vi "Main.vi"(8 "error in":errorcluster, 11 "Analog Signal in":refnum<class "Analog Signal.lvclass">) -> (0 "error out":errorcluster, 3 "Analog Signal out":refnum<class "Analog Signal.lvclass">)   [LabVIEW 2023, in "Analog Signal.lvclass"]
doc: "The <b>Queued Message Handler</b> of the Worker that owns this VI."
uses:
  Analog Signal.lvclass
  C:/Program Files (x86)/National Instruments/LabVIEW 2023/vi.lib/addons/_Workers/Library/Classes/Worker/Worker.lvclass
  Support/Signal Type.ctl
  Support/Signal Config.ctl
  Support/Sampling Config.ctl
  Initialization Data.ctl
  Response Cases.ctl
  <vilib>/addons/_Workers/Library/Case Label.ctl
  Analog Signal.lvclass/Analog Signal.ctl
  rql_Set Sampling Config.ctl
  rqp_Set Signal Config.ctl
  rqp_Set Sampling.ctl
  rqp_Insert to Subpanel.ctl
  rsp_Acquisition.ctl
  <vilib>/Utility/error.llb/Error Cluster From Error Code.vi
  <vilib>/ErrorRing/Error Ring.xnode
  Message Pump/Message Pump.lvclass
  <vilib>/addons/_Workers/Library/Workers.lvlib
panel:
  out "Response Cases.Sampling_Config":T1={"Fs"=1000.0, "#s"=1000.0} {"Fs" format="%.2p"}
  out "Response Cases.Signal_Config":T2={"offset"=0.0, "frequency"=10.0, "amplitude"=1.0} {"amplitude" format="%#_13g"; "frequency" format="%#_13g"; "offset" format="%0.2p"}
  out "Response Cases.Signal Type":T3
  out "Waveform Chart":waveform(dbl)(graph)
  # "Analog Signal"
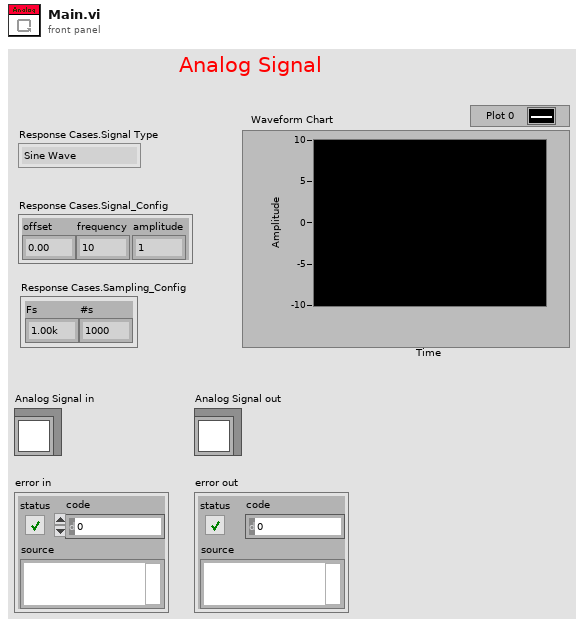
[diagram p1: front panel]
types:
  T1 = typedef "Analog Signal.lvclass/Sampling Config.ctl" = cluster{"Fs":dbl, "#s":dbl}
  T2 = typedef "Analog Signal.lvclass/Signal Config.ctl" = cluster{"offset":dbl, "frequency":dbl, "amplitude":dbl}
  T3 = typedef "Analog Signal.lvclass/Signal Type.ctl" = enum16{"Sine Wave", "Square Wave"}
  T4 = enum32{"Invalid", "Standard", "Closed", "Hidden", "Minimized", "Maximized"}
  T5 = typedef "Analog Signal.lvclass/Initialization Data.ctl" = cluster{"Response Cases":T6}
  T6 = typedef "Analog Signal.lvclass/Response Cases.ctl" = cluster{"Signal Type":T3, "Signal_Config":T2, "Sampling_Config":T1, "Acquisition":T7}
  T7 = typedef "Workers.lvlib/Case Label.ctl" = string
  T8 = typedef "Analog Signal.lvclass/rql_Set Sampling Config.ctl" = cluster{"Sampling_Config":T1}
  T9 = typedef "Analog Signal.lvclass/rqp_Set Signal Config.ctl" = cluster{"Signal_Config":T2, "Signal Type":T3}
  T10 = typedef "Analog Signal.lvclass/rqp_Set Sampling.ctl" = cluster{"Sampling_Config":T1}
  T11 = typedef "Analog Signal.lvclass/rqp_Insert to Subpanel.ctl" = cluster{"Sub Panel Ref":refnum<vi>}
  T12 = typedef "Analog Signal.lvclass/rsp_Acquisition.ctl" = cluster{"Waveform":waveform(dbl)}
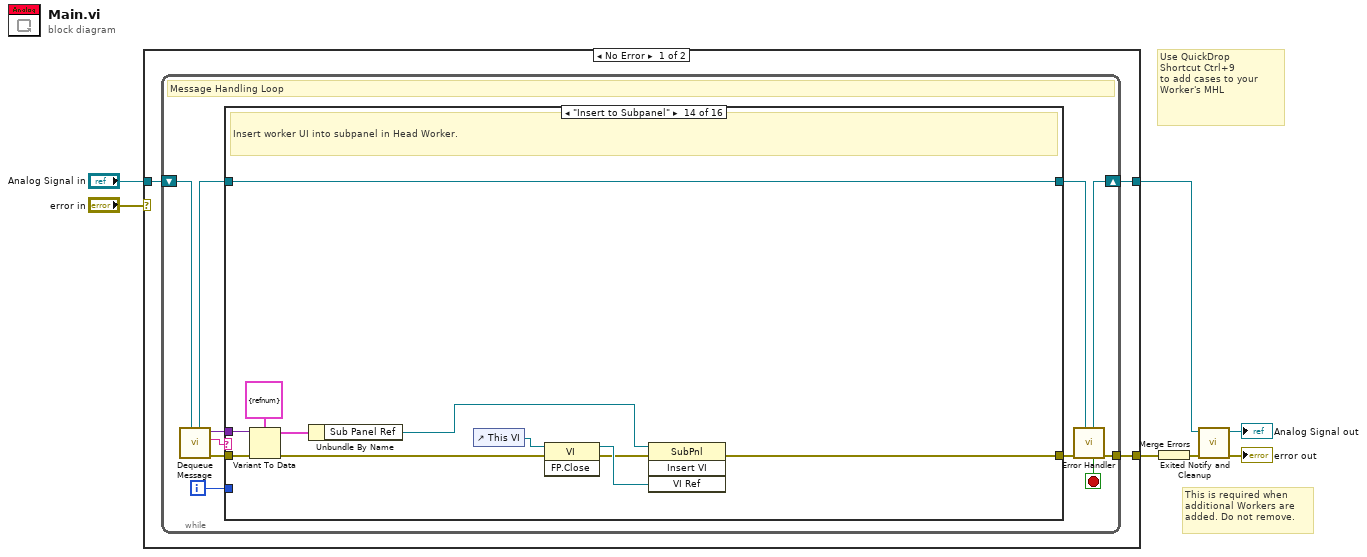
[diagram p0: block diagram]
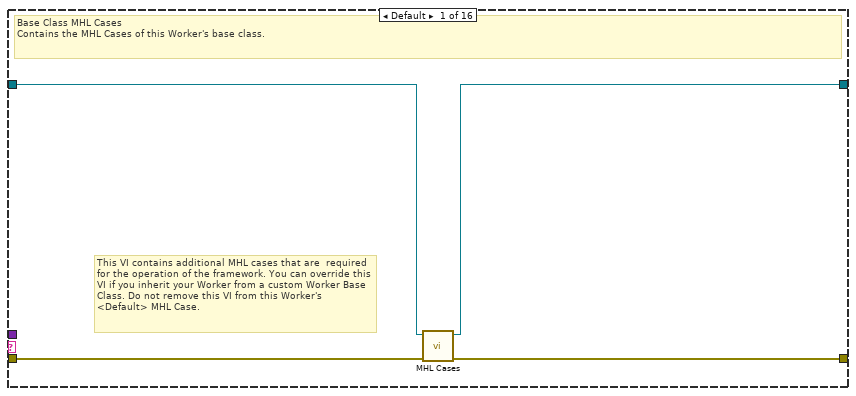
[diagram p2: hidden frame]
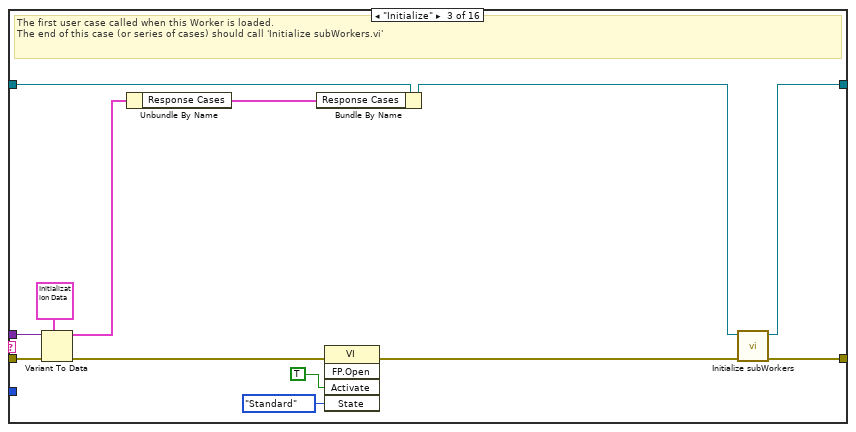
[diagram p4: hidden frame]
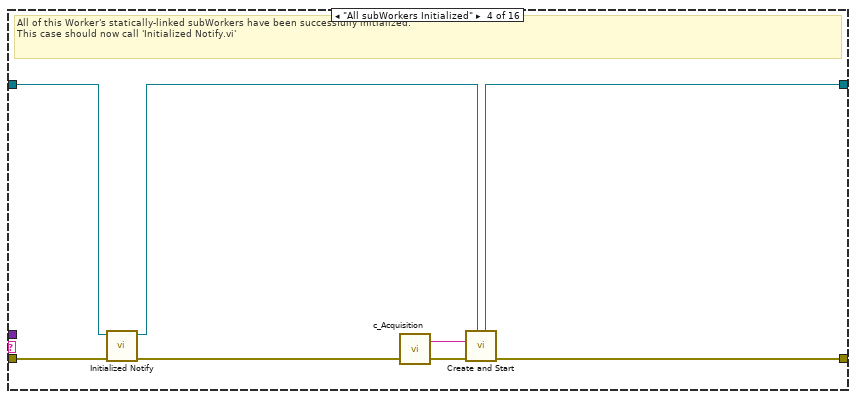
[diagram p5: hidden frame]
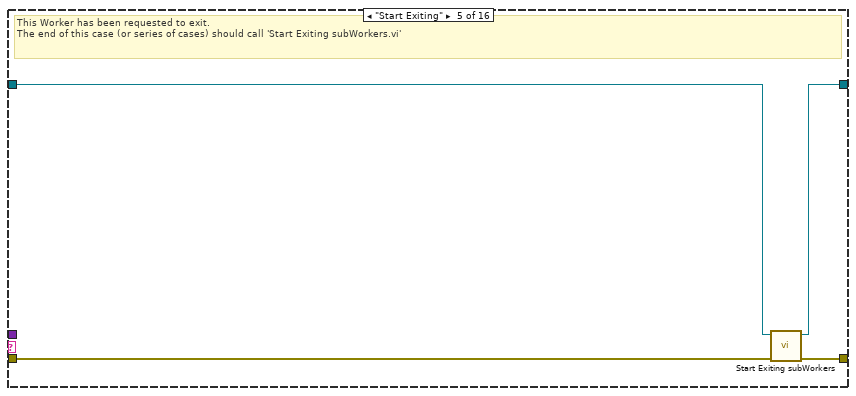
[diagram p6: hidden frame]
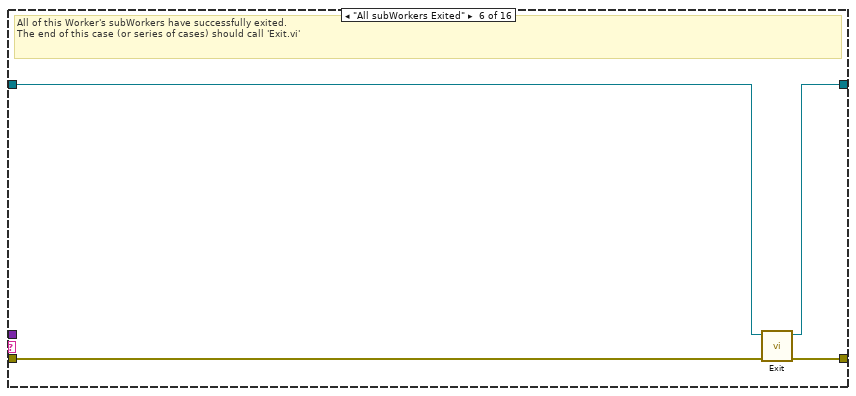
[diagram p7: hidden frame]
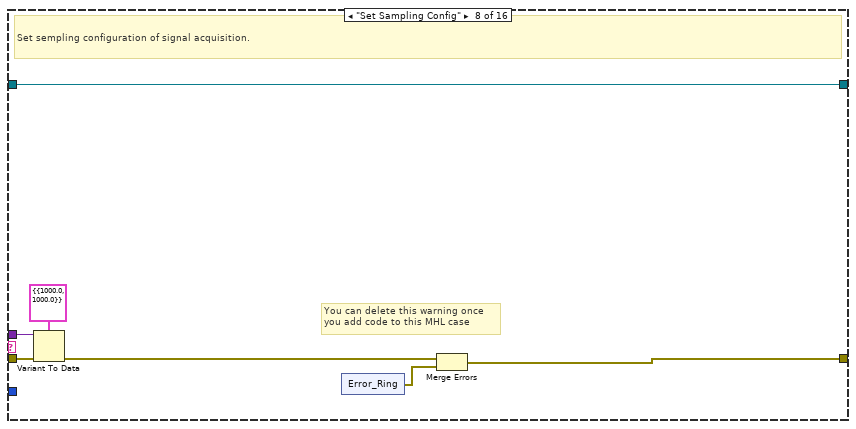
[diagram p9: hidden frame]
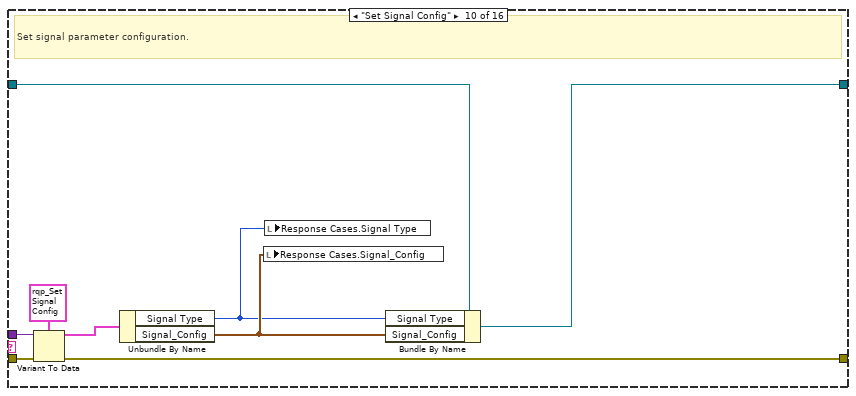
[diagram p11: hidden frame]
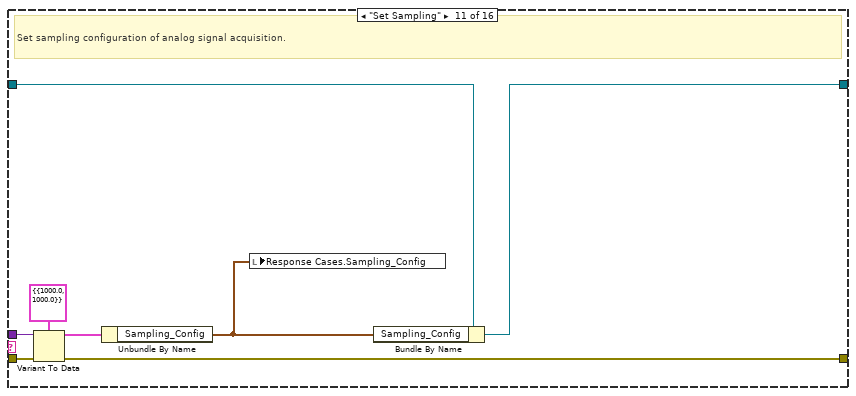
[diagram p12: hidden frame]
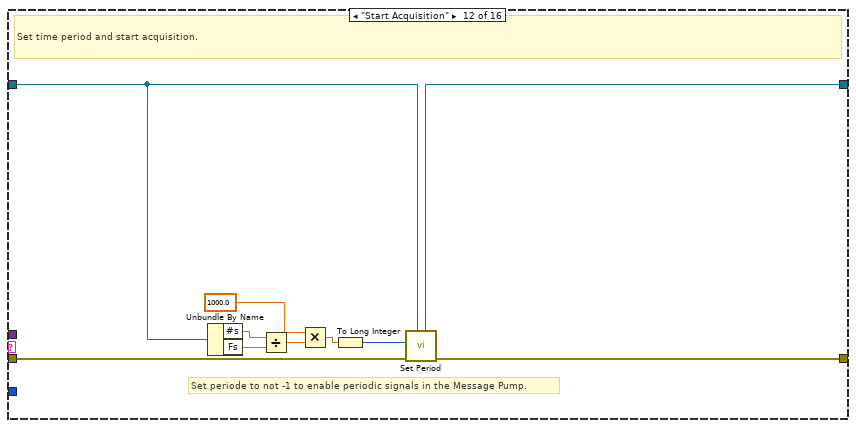
[diagram p13: hidden frame]
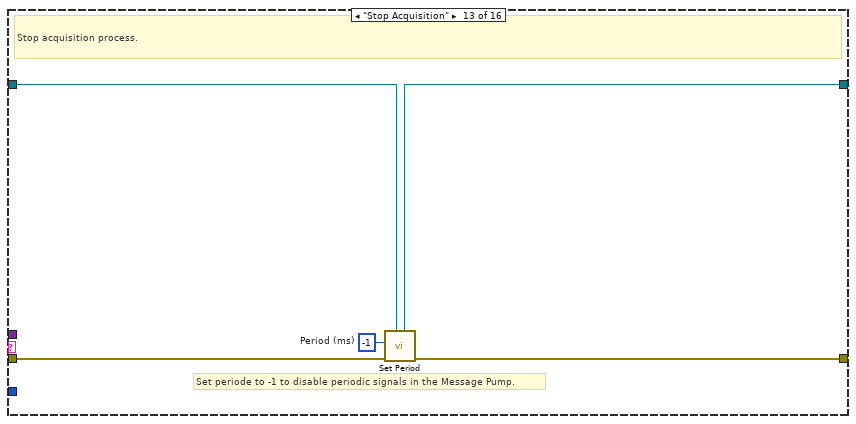
[diagram p14: hidden frame]
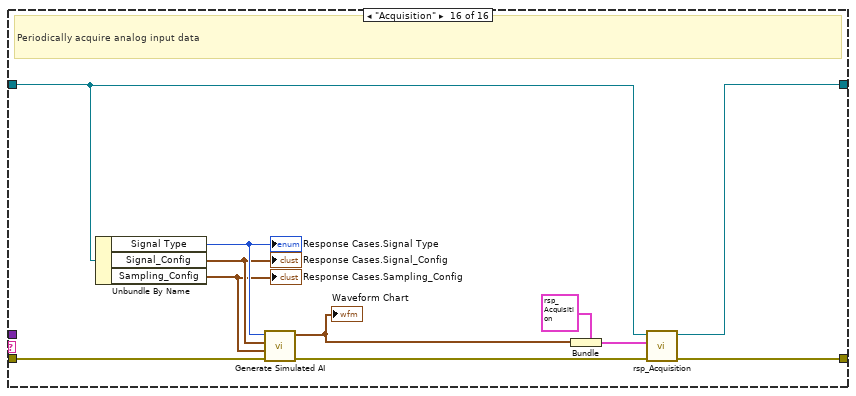
[diagram p16: hidden frame]
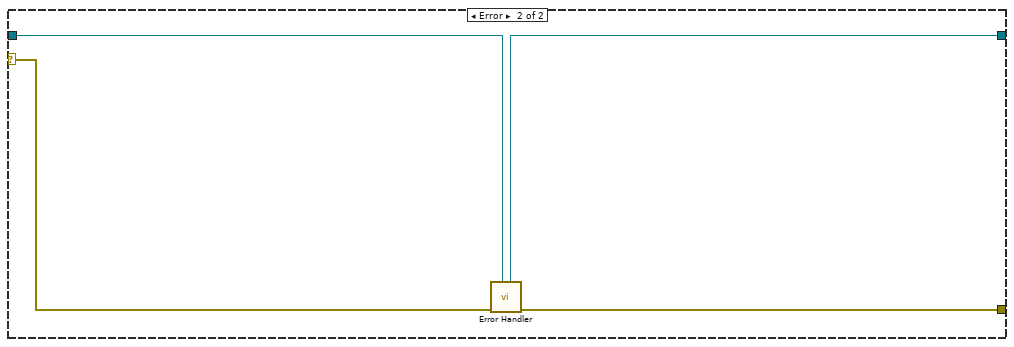
[diagram p17: hidden frame]
diagram:
  # "Use QuickDrop\nShortcut Ctrl+9\nto add cases to your\nWorker's MHL"
  # "This is required when additional Workers are added. Do not remove."
  n1 = case shown="No Error" "error in" {
    tunnel: "Analog Signal in" -> [w8 w129]
    tunnel: [w10 w130] -> w6
    tunnel: [w9 w128] -> w7
    selector: "error in" -> [_ w131]
    frame No Error {
      n2 = while {
        shift-right: [w19] -> w9
        shift-left: w8 -> [w21]
        tunnel: [w20] -> w10
        i -> [w12]
        stop <- w13 stop-if-true
        # "Message Handling Loop"
        n3 = call-dynamic "Dequeue Message.vi"("Worker"=w21) -> ("error out"=w18:errorcluster, "Case out"=w14:string, "Data out"=w11:variant, "Worker out"=w16:refnum<class "Analog Signal.lvclass">)  [unwired: 6 in, 1 out]
        n4 = case "Worker MHL Case Structure (DO NOT CHANGE LABEL NAME)" shown="\"Insert to Subpanel\"" w14 {
          tunnel: w18 -> [w25 w26 w38 w47 w48 w55 w57 w63 w71 w79 w88 w97 w100 w113 w116 w127]
          tunnel: [w24 w26 w40 w42 w51 w54 w57 w59 w71 w78 w87 w96 w99 w104 w116 w122] -> w17
          tunnel: w16 -> [w23 w27 w37 w46 w49 w53 w56 w64 w70 w80 w84 w95 w102 w114 w115 w121]
          tunnel: [w22 w27 w39 w44 w50 w52 w56 w64 w70 w75 w83 w98 w101 w114 w115 w120] -> w15
          tunnel: w12 -> [_ _ _ _ _ _ _ _ _ _ _ _ _ _ _ _]
          tunnel: w11 -> [_ _ w36 _ _ _ _ w60 _ w76 w85 _ _ w111 _ _]
          frame Default {
            # "This VI contains additional MHL cases that are  required for the operation of the framework. You can override this VI if you inherit your Worker from a custom Worker Base Class. Do not remove this VI from this Worker's <Default> MHL Case."
            # "Base Class MHL Cases\nContains the MHL Cases of this Worker's base class."
            n5 = call-dynamic "MHL Cases.vi"("error in"=w25, "Worker in"=w23) -> ("error out"=w24:errorcluster, "Worker out"=w22:refnum<class "Analog Signal.lvclass">)  [unwired: 8 in]
          }
          frame "------------ FRAMEWORK CASES -----------" {
            # "Start of Workers Framework Cases"
          }
          frame "Initialize" {
            # "The first user case called when this Worker is loaded.\nThe end of this case (or series of cases) should call 'Initialize subWorkers.vi'"
            n6 = Variant To Data(error in=w38, type=T5 {"Response Cases"={"Signal Type"=enum."Sine Wave", "Signal_Config"={"offset"=0.0, "frequency"=10.0, "amplitude"=1.0}, "Sampling_Config"={"Fs"=1000.0, "#s"=1000.0}, "Acquisition"=""}} ("Cluster"), Variant=w36) -> (data=w34:T5, error out=w29:errorcluster)
            n7 = Unbundle By Name(w34) -> ("Response Cases"=w33:T6)
            n8 = Bundle By Name(cluster=w37, "Response Cases"=w33) -> (w35:refnum<class "Analog Signal.lvclass">)
            n9 = invoke class="VI" method="FP.Open"(error in=w29, "Activate"=TRUE ("Activate?"), "State"=T4."Standard") -> (error out=w28:errorcluster)  [unwired: 2 in, 4 out]
            n10 = call-dynamic "Initialize subWorkers.vi"("error in"=w28, "Worker"=w35) -> ("error out"=w40:errorcluster, "dup Worker out"=w39:refnum<class "Analog Signal.lvclass">)  [unwired: 8 in]
          }
          frame "All subWorkers Initialized" {
            # "All of this Worker's statically-linked subWorkers have been successfully initialized.\nThis case should now call 'Initialized Notify.vi'"
            n11 = call-dynamic "Initialized Notify.vi"("error in"=w47, "Worker"=w46) -> ("error out"=w43:errorcluster, "dup Worker out"=w45:refnum<class "Analog Signal.lvclass">)  [unwired: 8 in]
            n12 = call "c_Acquisition.vi"() -> ("Case Label"=w41:T7)  [unwired: 1 in]
            n13 = call "Create and Start.vi"("Caller"=w45, "error in (no error)"=w43, "Time Elapsed Response Case (Case Label)"=w41) -> ("error out"=w42:errorcluster, "dup Caller out"=w44:refnum<class "Analog Signal.lvclass">)  [unwired: 6 in, 1 out]
          }
          frame "Start Exiting" {
            # "This Worker has been requested to exit. \nThe end of this case (or series of cases) should call 'Start Exiting subWorkers.vi'"
            n14 = call-dynamic "Start Exiting subWorkers.vi"("error_in"=w48, "Worker"=w49) -> ("error out"=w51:errorcluster, "dup Worker out"=w50:refnum<class "Analog Signal.lvclass">)  [unwired: 8 in]
          }
          frame "All subWorkers Exited" {
            # "All of this Worker's subWorkers have successfully exited. \nThe end of this case (or series of cases) should call 'Exit.vi'"
            n15 = call-dynamic "Exit.vi"("error_in"=w55, "Worker"=w53) -> ("error out"=w54:errorcluster, "dup Worker out"=w52:refnum<class "Analog Signal.lvclass">)  [unwired: 8 in]
          }
          frame "------------- LOCAL API CASES -------------" {
            # "Start of Workers Local API Cases"
          }
          frame "Set Sampling Config" {
            # "You can delete this warning once\nyou add code to this MHL case"
            # "Set sempling configuration of signal acquisition."
            n16 = Variant To Data(error in=w63, type=T8 {"Sampling_Config"={"Fs"=1000.0, "#s"=1000.0}} ("Data"), Variant=w60) -> (error out=w62:errorcluster)  [unwired: 1 out]
            n17 = xnode ("Error_Ring")() -> ("error out"=w58:errorcluster)
            n18 = Merge Errors(w62, w58) -> (w59:errorcluster)
          }
          frame "------------- PUBLIC API CASES -------------" {
            # "Start of Workers Public API Cases"
          }
          frame "Set Signal Config" {
            # "Set signal parameter configuration."
            n19 = Variant To Data(error in=w79, type=T9 {"Signal_Config"={"offset"=0.0, "frequency"=10.0, "amplitude"=1.0}, "Signal Type"=enum."Sine Wave"} ("Data"), Variant=w76) -> (data=w74:T9, error out=w78:errorcluster)
            n20 = Unbundle By Name(w74) -> ("Signal Type"=w72:T3, "Signal_Config"=w73:T2)
            n21 = local write "Response Cases.Signal_Config"(w73) -> ()
            n22 = local write "Response Cases.Signal Type"(w72) -> ()
            n23 = Bundle By Name(cluster=w80, "Signal Type"=w72, "Signal_Config"=w73) -> (w75:refnum<class "Analog Signal.lvclass">)
          }
          frame "Set Sampling" {
            # "Set sampling configuration of analog signal acquisition."
            n24 = Variant To Data(error in=w88, type=T10 {"Sampling_Config"={"Fs"=1000.0, "#s"=1000.0}} ("Data"), Variant=w85) -> (data=w82:T10, error out=w87:errorcluster)
            n25 = Unbundle By Name(w82) -> ("Sampling_Config"=w81:T1)
            n26 = local write "Response Cases.Sampling_Config"(w81) -> ()
            n27 = Bundle By Name(cluster=w84, "Sampling_Config"=w81) -> (w83:refnum<class "Analog Signal.lvclass">)
          }
          frame "Start Acquisition" {
            # "Set periode to not -1 to enable periodic signals in the Message Pump."
            # "Set time period and start acquisition."
            n28 = Unbundle By Name(w95) -> ("#s"=w94:dbl, "Fs"=w93:dbl)
            n29 = Divide(x=w94, y=w93) -> (x/y=w91:dbl)
            n30 = Multiply(x=1000.0, y=w91) -> (x*y=w90:dbl)
            n31 = To Long Integer(number=w90) -> (32bit integer=w92:i32)
            n32 = call "Set Period.vi"("Caller"=w95, "error in"=w97, "Period (ms)"=w92) -> ("error out"=w96:errorcluster, "dup Caller out"=w98:refnum<class "Analog Signal.lvclass">)  [unwired: 7 in]
          }
          frame "Stop Acquisition" {
            w103 = -1  # Period (ms)
            # "Set periode to -1 to disable periodic signals in the Message Pump."
            # "Stop acquisition process."
            n33 = call "Set Period.vi"("Caller"=w102, "error in"=w100, "Period (ms)"=w103) -> ("error out"=w99:errorcluster, "dup Caller out"=w101:refnum<class "Analog Signal.lvclass">)  [unwired: 7 in]
          }
          frame "Insert to Subpanel" {
            # "Insert worker UI into subpanel in Head Worker."
            n34 = Variant To Data(error in=w113, type=T11 {"Sub Panel Ref"=refnum} ("Data"), Variant=w111) -> (data=w110:T11, error out=w105:errorcluster)
            n35 = Unbundle By Name(w110) -> ("Sub Panel Ref"=w108:refnum<vi>)
            n36 = control-ref of="This VI"() -> (w109:refnum<vi>)
            n37 = invoke class="VI" method="FP.Close"(reference=w109, error in=w105) -> (reference out=w107:refnum<vi>, error out=w106:errorcluster)  [unwired: 1 in, 1 out]
            n38 = invoke class="SubPnl" method="Insert VI"(reference=w108, error in=w106, "VI Ref"=w107) -> (error out=w104:errorcluster)  [unwired: 1 in, 3 out]
          }
          frame "------------- RESPONSE CASES --------------" {
            # "Start of Workers Response Cases"
          }
          frame "Acquisition" {
            # "Periodically acquire analog input data"
            n39 = Unbundle By Name(w121) -> ("Signal Type"=w126:T3, "Signal_Config"=w125:T2, "Sampling_Config"=w124:T1)
            "Response Cases.Signal Type" <- w126
            "Response Cases.Signal_Config" <- w125
            "Response Cases.Sampling_Config" <- w124
            n40 = call "Generate Simulated AI.vi"("error in (no error)"=w127, "Sampling_Config"=w124, "Signal_Config"=w125, "Signal Type"=w126) -> ("error out"=w123:errorcluster, "Graph Data"=w117:waveform(dbl))  [unwired: 6 in]
            "Waveform Chart" <- w117
            n41 = Bundle(cluster=T12 {"Waveform"={"t0"=timestamp(0 s since 1904-01-01), "dt"=1.0, "Y"=[]}} ("Data in"), "Waveform"=w117) -> (w118:T12)
            n42 = call "rsp_Acquisition.vi"("error in"=w123, "Data in"=w118, "Analog Signal in"=w121) -> ("error out"=w122:errorcluster, "dup Analog Signal out"=w120:refnum<class "Analog Signal.lvclass">)  [unwired: 7 in]
          }
        }
        n43 = call-dynamic "Error Handler.vi"("Worker"=w15, "error_in"=w17) -> ("error out"=w20:errorcluster, "Stop Loop"=w13:bool, "Worker out"=w19:refnum<class "Analog Signal.lvclass">)  [unwired: 7 in]
      }
    }
    frame Error {
      n44 = call-dynamic "Error Handler.vi"("Worker"=w129, "error_in"=w131) -> ("error out"=w130:errorcluster, "Worker out"=w128:refnum<class "Analog Signal.lvclass">)  [unwired: 7 in, 1 out]
    }
  }
  n45 = Merge Errors(w6) -> (w3:errorcluster)
  n46 = call-dynamic "Exited Notify and Cleanup.vi"("error_in"=w3, "Worker"=w7) -> ("error out"=→"error out":errorcluster, "dup Worker out"=→"Analog Signal out":refnum<class "Analog Signal.lvclass">)  [unwired: 8 in]
